vi "hextoword.vi"(0 "object in":refnum<class "interface.lvclass">, 1 "数组":u16[](array[numeric]) format="%04xH", 5 "error in (no error)":errorcluster) -> (14 "object out":refnum<class "interface.lvclass">, 15 "WORD":u16[](array[numeric]), 19 "error out":errorcluster)   [LabVIEW 2016, in "interface.lvclass"]
uses:
  interface.lvclass
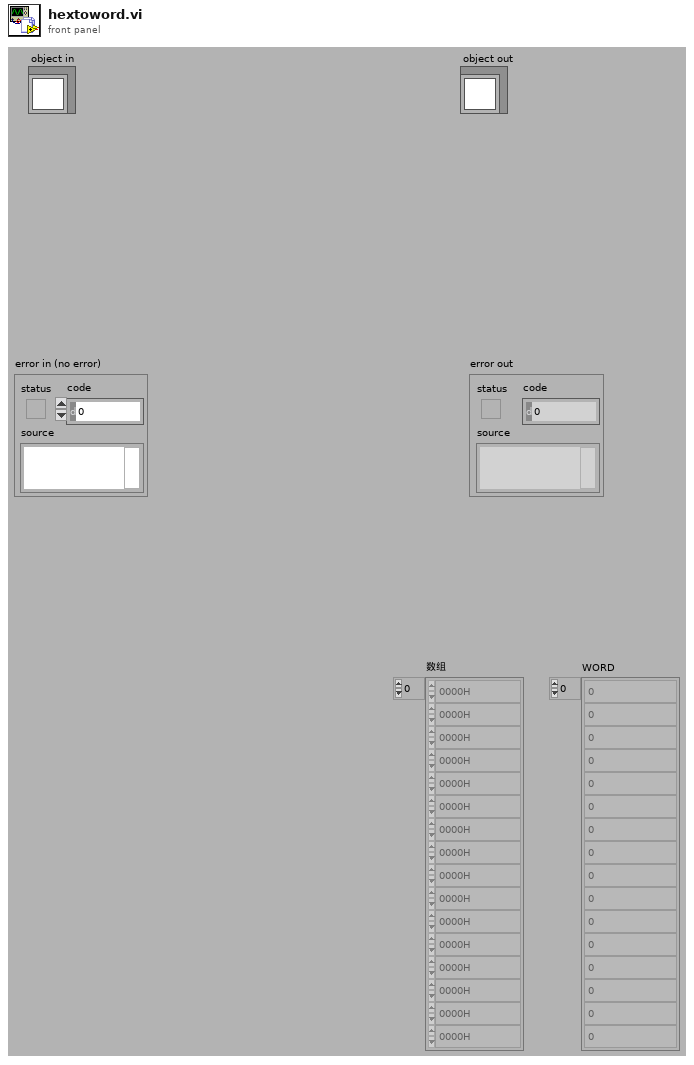
[diagram p1: front panel]
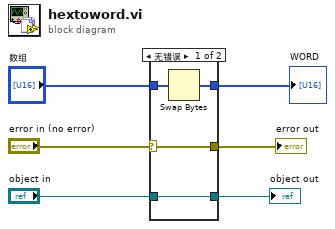
[diagram p0: block diagram]
diagram:
  n1 = case shown="无错误" "error in (no error)" {
    selector: "error in (no error)" -> [w10 w12]
    tunnel: [w10 w12] -> w5
    tunnel: [w9 w11] -> w3
    tunnel: "object in" -> [w9 w11]
    tunnel: "数组" -> [w8 _]
    tunnel: [w7 _] -> w1
    frame No Error {
      n2 = Swap Bytes(anything=w8) -> (byte swapped=w7:u16[])
    }
    frame Error {
    }
  }
  "error out" <- w5
  "object out" <- w3
  "WORD" <- w1
